vi "InitializeSubVI2.vi"(0 "Exposure Time (secs)":sgl format="%.2f") -> (1 "Initialize (bool 1)":bool, 2 "Set image (bool 2)":bool, 3 "Check timings (bool 3)":bool)   [LabVIEW 2019]
uses:
  atmcd32d.dll
panel:
  out "Set Image":u32
  out "Set Gate Mode":u32
  out "Detector Y Pixels":i32
  out "Get Detector":u32
  out "Set Exposure Time":u32
  out "Set Trigger Mode":u32
  out "Set Readout Mode":u32
  out "Set Acquisition Mode":u32
  out "Check Timings":u32
  out "Detector X Pixels":i32
  out "Calculated Exposure Value":sgl format="%.5f"
  out "Initialize":u32
  in  "Trigger":u32(ring) items=["Internal", "External"]
  # "Status"
  # "Return values"
  # "USB iStarIMAG32at.VI"
  # "Acquisition Mode: Single Scan\nReadout Mode: Full Resolution Image"
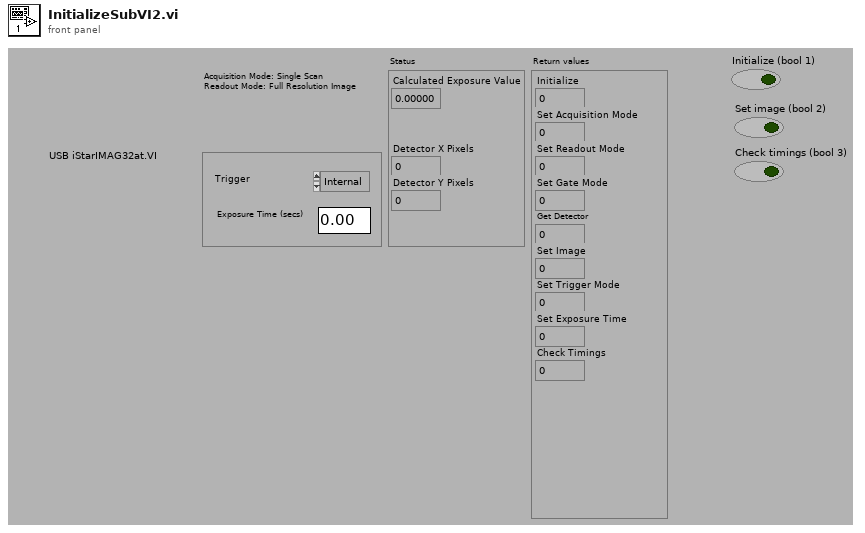
[diagram p1: front panel]
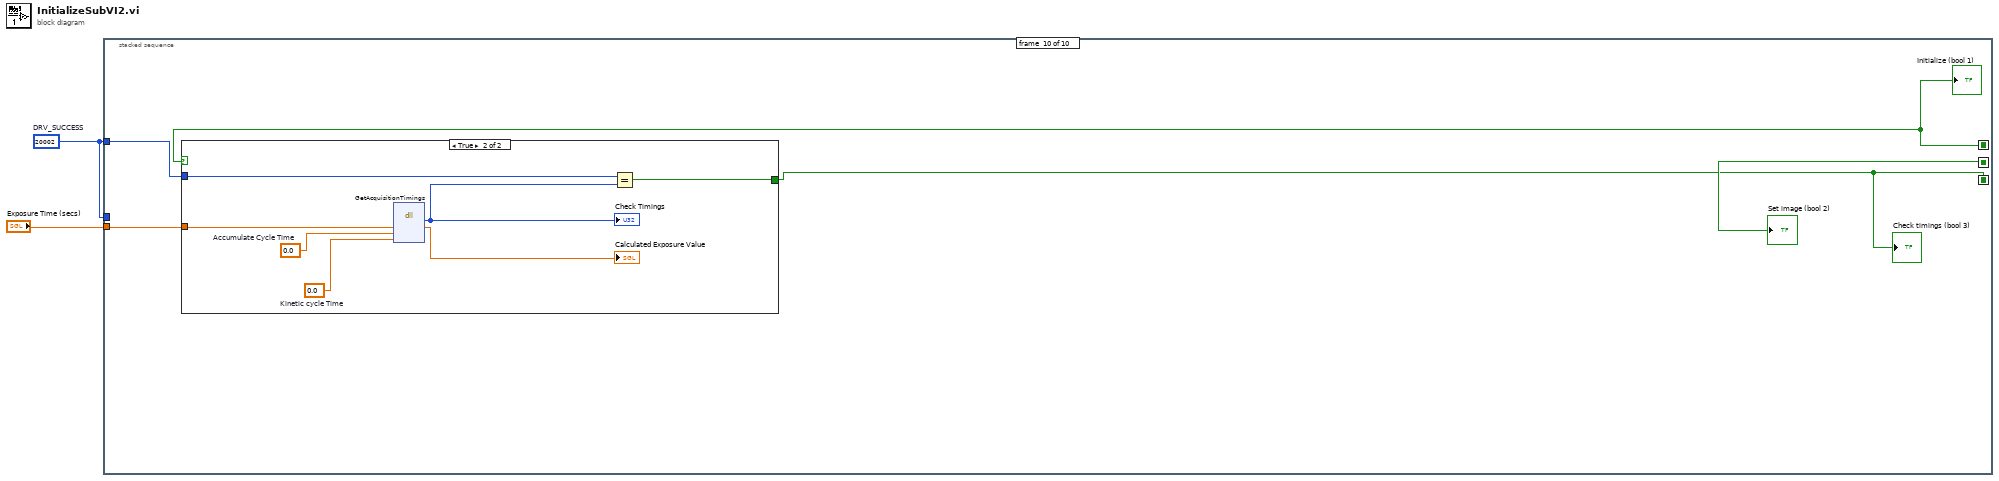
[diagram p0: block diagram]
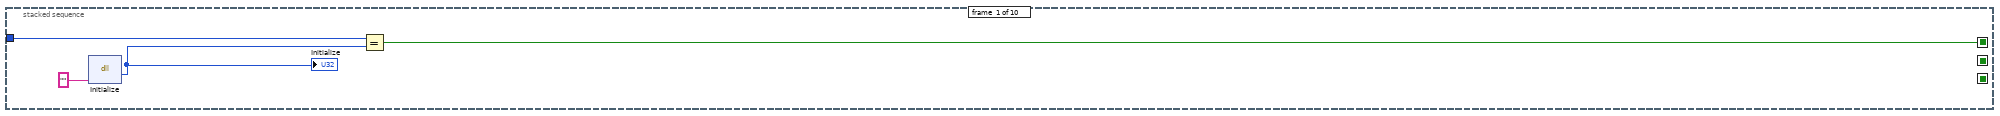
[diagram p2: hidden frame]
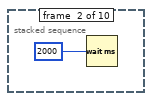
[diagram p3: hidden frame]
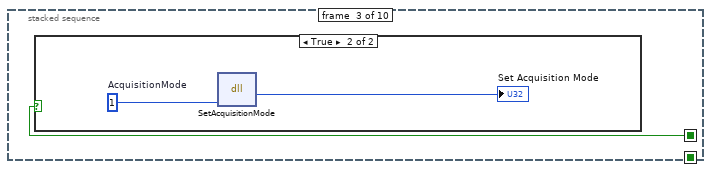
[diagram p4: hidden frame]
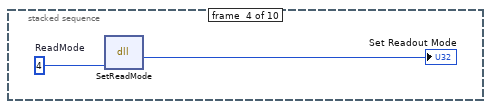
[diagram p6: hidden frame]
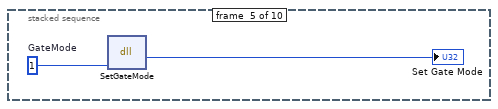
[diagram p7: hidden frame]
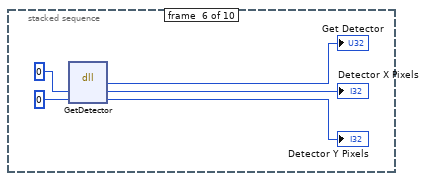
[diagram p8: hidden frame]
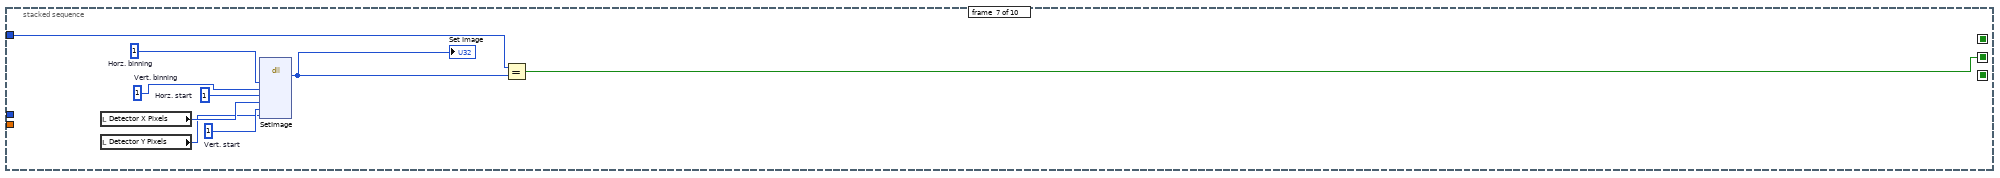
[diagram p9: hidden frame]
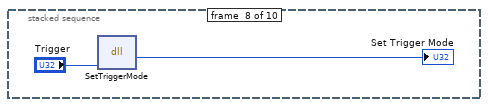
[diagram p10: hidden frame]
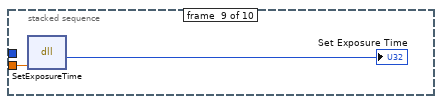
[diagram p11: hidden frame]
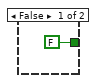
[diagram p12: hidden frame]
diagram:
  w1 = 20002  # DRV_SUCCESS
  n1 = stacked-sequence {
    seq-local: [w4 _ _ _ _ _ _ _ _ _] -> [_ _ w8 _ _ _ _ _ _ w35]
    seq-local: [_ _ _ _ _ _ _ _ _ w33] -> [_ _ _ _ _ _ _ _ _ _]
    seq-local: [_ _ _ _ _ _ w20 _ _ _] -> [_ _ _ _ _ _ _ _ _ w34]
    tunnel: "Exposure Time (secs)" -> [_ _ _ _ _ _ _ _ w32 w37]
    tunnel: w1 -> [w5 _ _ _ _ _ w22 _ _ w36]
    tunnel: w1 -> [_ _ _ _ _ _ _ _ _ _]
    frame #0 {
      n2 = dll-call lib="atmcd32d.dll" fn="Initialize" label="Call Library Function Initialize"("") -> (w6:u32)  [unwired: 4 in, 2 out]
      "Initialize" <- w6
      n3 = Equal?(x=w5, y=w6) -> (x = y?=w4:bool)
    }
    frame #1 {
      n4 = Wait (ms)(milliseconds to wait=u32 2000) -> ()  [unwired: 1 out]
    }
    frame #2 {
      n5 = case shown="True" w8 {
        frame False {
        }
        frame True {
          w10 = u16 1  # AcquisitionMode
          n6 = dll-call lib="atmcd32d.dll" fn="SetAcquisitionMode" label="Call Library Function SetAcquisitionMode"(w10) -> (→"Set Acquisition Mode":u32)  [unwired: 4 in, 2 out]
        }
      }
    }
    frame #3 {
      w12 = u16 4  # ReadMode
      n7 = dll-call lib="atmcd32d.dll" fn="SetReadMode" label="Call Library Function SetReadMode"(w12) -> (→"Set Readout Mode":u32)  [unwired: 4 in, 2 out]
    }
    frame #4 {
      w14 = u16 1  # GateMode
      n8 = dll-call lib="atmcd32d.dll" fn="SetGateMode" label="Call Library Function SetGateMode"(w14) -> (→"Set Gate Mode":u32)  [unwired: 4 in, 2 out]
    }
    frame #5 {
      n9 = dll-call lib="atmcd32d.dll" fn="GetDetector" label="Call Library FunctionGetDetector"(i16 0, i16 0) -> (→"Get Detector":u32, →"Detector X Pixels":i32, →"Detector Y Pixels":i32)  [unwired: 3 in, 2 out]
    }
    frame #6 {
      w25 = u16 1  # Vert. start
      w26 = u16 1  # Horz. start
      w27 = u16 1  # Vert. binning
      w28 = u16 1  # Horz. binning
      n10 = local read "Detector X Pixels"() -> (w24:i32)
      n11 = local read "Detector Y Pixels"() -> (w23:i32)
      n12 = dll-call lib="atmcd32d.dll" fn="SetImage" label="Call Library Function SetImage"(w28, w27, w26, w24, w25, w23) -> (w21:u32)  [unwired: 9 in, 2 out]
      "Set Image" <- w21
      n13 = Equal?(x=w22, y=w21) -> (x = y?=w20:bool)
    }
    frame #7 {
      n14 = dll-call lib="atmcd32d.dll" fn="SetTriggerMode" label="Call Library Function SetTrigger Mode"("Trigger") -> (→"Set Trigger Mode":u32)  [unwired: 4 in, 2 out]
    }
    frame #8 {
      n15 = dll-call lib="atmcd32d.dll" fn="SetExposureTime" label="Call Library FunctionSet Exposure Time"(w32) -> (→"Set Exposure Time":u32)  [unwired: 4 in, 2 out]
    }
    frame #9 {
      n16 = case shown="True" w35 {
        tunnel: w37 -> [_ w42]
        tunnel: w36 -> [_ w39]
        tunnel: [FALSE w41] -> w33
        frame False {
        }
        frame True {
          w44 = sgl 0.0  # Accumulate Cycle Time
          w45 = sgl 0.0  # Kinetic cycle Time
          n17 = dll-call lib="atmcd32d.dll" fn="GetAcquisitionTimings" label="Call Library Function Check Timings"(w42, w44, w45) -> (w40:u32, →"Calculated Exposure Value":sgl)  [unwired: 5 in, 2 out]
          "Check Timings" <- w40
          n18 = Equal?(x=w39, y=w40) -> (x = y?=w41:bool)
        }
      }
      "Check timings (bool 3)" <- w33
      "Initialize (bool 1)" <- w35
      "Set image (bool 2)" <- w34
    }
  }
